vi "Initialize UUDT Database.vi"(8 "error in (no error)":errorcluster, 10 "Baud Rate":u32, 11 "Addon Name":string) -> (0 "error out":errorcluster, 2 "Cluster":refnum<k21>, 3 "XNET Database":refnum<k21>)   [LabVIEW 2015, in "GMLAN.lvlib"]
uses:
  GMLAN.lvlib
  <vilib>/xnet/xnet.llb/XNET Database Open (Database).vi
  <resource>/objmgr/xnet.rc
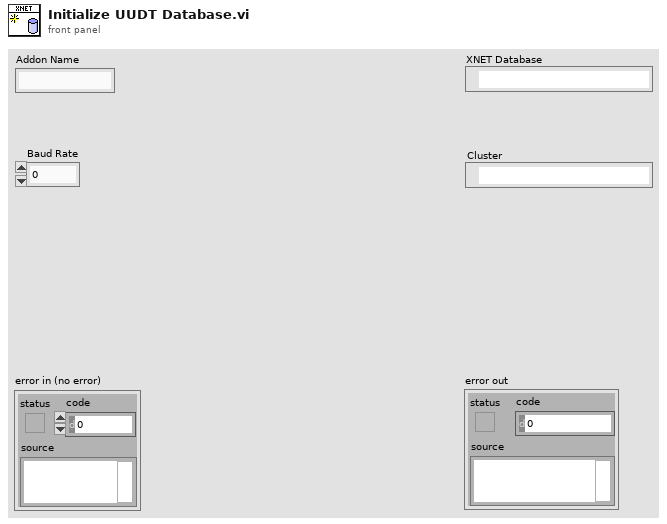
[diagram p1: front panel]
types:
  T1 = cluster{"Baud Rate":u32, "Comment":string, "Name":string}
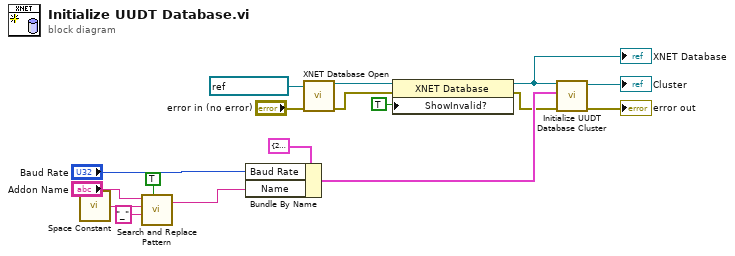
[diagram p0: block diagram]
diagram:
  n1 = call <vilib>:"Space Constant.vi"() -> ("String"=w8:string)
  n2 = call <vilib>:"Search and Replace Pattern.vi"("string"="Addon Name", "regular expression (\"\")"=w8, "replace string (\"\")"="_" ("replace string (\"\")"), "replace all? (F)"=TRUE) -> ("result string"=w6:string)  [unwired: 1 in, 1 out]
  n3 = Bundle By Name(cluster=T1 {"Baud Rate"=250000, "Comment"="", "Name"="UUDT"} ("CAN Cluster"), "Baud Rate"="Baud Rate", "Name"=w6) -> (w15:T1)
  n4 = call-poly <vilib>:"XNET Database Open.vi"("database in (:memory:)"=refnum<k21> ":memory:", "error in (no error)"="error in (no error)") -> ("database out"=w12:refnum<k21>, "error out"=w4:errorcluster)  [unwired: 12 out]
  n5 = property class="XNET Database"(reference=w12, error in=w4, "ShowInvalid?"=TRUE ("Show Invalid From Open?")) -> (reference out=w5:refnum<k21>, error out=w3:errorcluster)
  "XNET Database" <- w5
  n6 = call "Initialize UUDT Database Cluster.vi"("error in"=w3, "CAN Cluster"=w15, "database in"=w5) -> ("error out"=→"error out":errorcluster, "cluster out"=→"Cluster":refnum<k21>)  [unwired: 7 out]
